vi "KE622x -- Delta Mode Get Num Cycles.vi"(0 "Resource In":refnum<visa-resource-name>, 1 "Check For SCPI Errors? (T)":bool=TRUE, 11 "error in (no error)":errorcluster) -> (4 "Resource Out (dupl)":refnum<visa-resource-name>, 6 "Num Cycles Mode":T1, 8 "Finite Count":T2=1 min=1 max=65536, 15 "error out":errorcluster)   [LabVIEW 2020, in "Keithley 622x.lvlib"]
uses:
  Keithley 622x.lvlib
  Typedefs/KE622x -- Delta PDelta Mode Num Cycles.ctl
  Typedefs/KE622x -- Delta PDelta Mode Num Cycles Mode.ctl
panel:
  # "*** NOTE:  \"Finite Count\" is only valid\nif \"Num Cycles Mode\" is 'Finite Count'."
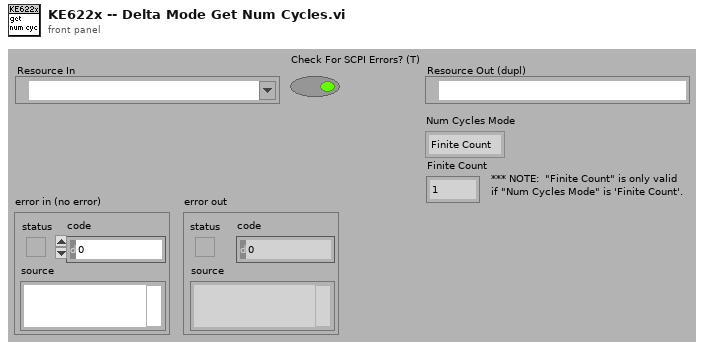
[diagram p1: front panel]
types:
  T1 = typedef "Keithley 622x.lvlib/KE622x -- Delta PDelta Mode Num Cycles Mode.ctl" = enum16{"Finite Count", "Infinite"}
  T2 = typedef "Keithley 622x.lvlib/KE622x -- Delta PDelta Mode Num Cycles.ctl" = u32
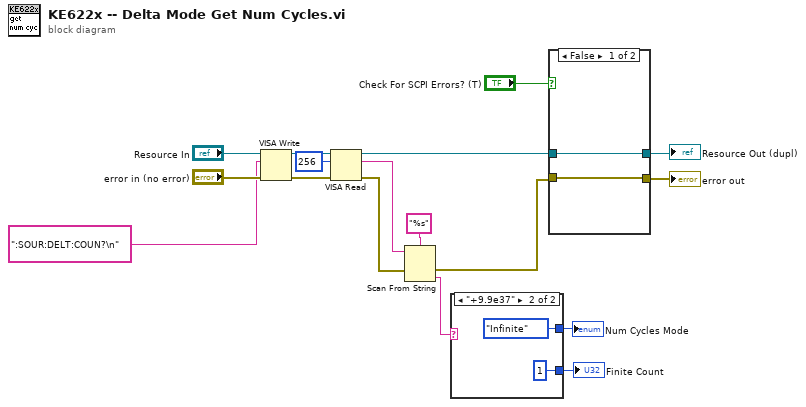
[diagram p0: block diagram]
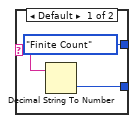
[diagram p2: hidden frame]
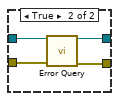
[diagram p3: hidden frame]
diagram:
  n1 = VISA Write(VISA resource name="Resource In", write buffer=":SOUR:DELT:COUN?\n" ("format string"), error in (no error)="error in (no error)") -> (VISA resource name out=w11:refnum<visa-resource-name>, error out=w10:errorcluster)  [unwired: 1 out]
  n2 = VISA Read(VISA resource name=w11, byte count=u32 256, error in (no error)=w10) -> (VISA resource name out=w4:refnum<visa-resource-name>, read buffer=w6:string, error out=w8:errorcluster)  [unwired: 1 out]
  n3 = Scan From String(format string="%s", input string=w6, error in=w8) -> (error out=w5:errorcluster, output 1=w3:string)  [unwired: 2 in, 2 out]
  n4 = case shown="\"+9.9e37\"" w3 {
    selector: w3 -> [w19 _]
    tunnel: [KE622x_--_Delta_PDelta_Mode_Num_Cycles_Mode."Finite Count" ("Num Cycles Mode") KE622x_--_Delta_PDelta_Mode_Num_Cycles_Mode."Infinite" ("Num Cycles Mode")] -> w2
    tunnel: [w18 1] -> w1
    frame Default {
      n5 = Decimal String To Number(string=w19) -> (number=w18:i32)  [unwired: 2 in, 1 out]
    }
    frame "+9.9e37" {
    }
  }
  "Finite Count" <- w1
  "Num Cycles Mode" <- w2
  n6 = case shown="False" "Check For SCPI Errors? (T)" {
    tunnel: w4 -> [w24 w28]
    tunnel: w5 -> [w23 w27]
    tunnel: [w23 w26] -> w13
    tunnel: [w24 w25] -> w14
    frame False {
    }
    frame True {
      n7 = call "Error Query.vi"("VISA Resource In"=w28, "error in (no error)"=w27) -> ("VISA Resource Out (dupl)"=w25:refnum<visa-resource-name>, "error out"=w26:errorcluster)  [unwired: 10 in, 2 out]
    }
  }
  "Resource Out (dupl)" <- w14
  "error out" <- w13
